vi "data_type_equal.vi"(8 "error in":errorcluster, 10 "Data Cluster":variant, 11 "Stream data cluster":refnum<class "stream_custom_cluster.lvclass">) -> (0 "error out":errorcluster, 2 "dub Data Cluster":variant, 3 "Stream data cluster out":refnum<class "stream_custom_cluster.lvclass">)   [LabVIEW 2020, in "stream_custom_cluster.lvclass"]
uses:
  stream_custom_cluster.lvclass
  stream_custom_cluster.lvclass/stream_custom_cluster.ctl
  <vilib>/Utility/Data Type/NI_Data Type.lvlib
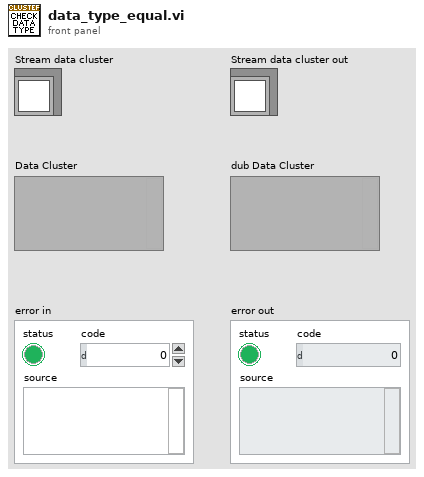
[diagram p1: front panel]
types:
  T1 = typedef "stream_custom_cluster.lvclass/private data.ctl" = cluster{"type":T2[], "channel names":string[], "data":refnum<queue>[], "cluster element types":variant[]}
  T2 = typedef "openg_variant.lvlib/Type Descriptor Enumeration__ogtk.ctl" = enum8{"<Null>", "I8", "I16", "I32", "I64", "U8", "U16", "U32", "U64", "SGL", "DBL", "EXT", "CSG", "CDB", "CXT", "0x0F", "0x10", "0x11", "0x12", "0x13", "0x14", "Enum U8", "Enum U16", "Enum U32", "Enum U64", "SGL PQ", "DBL PQ", "EXT PQ", "CSG PQ", "CDB PQ", "CXT PQ", "0x1F", "0x20", "Boolean", "0x22", "0x23", "0x24", "0x25", "0x26", "0x27", "0x28", "0x29", "0x2A", "0x2B", "0x2C", "0x2D", "0x2E", "0x2F", "String", "0x31", "Path", "Pict", "0x34", "0x35", "0x36", "DAQ", "0x38", "0x39", "0x3A", "0x3B", "0x3C", "0x3D", "0x3E", "0x3F", "Array", "0x41", "0x42", "0x43", "0x44", "0x45", "0x46", "0x47", "0x48", "0x49", "0x4A", "0x4B", "0x4C", "0x4D", "0x4E", "0x4F", "Cluster", "0x51", "0x52", "Variant", "Waveform", "0x55", "0x56", "0x57", "0x58", "0x59", "0x5A", "0x5B", "0x5C", "0x5D", "0x5E", "Fixed Point", "0x60", "0x61", "0x62", "0x63", "0x64", "0x65", "0x66", "0x67", "0x68", "0x69", "0x6A", "0x6B", "0x6C", "0x6D", "0x6E", "0x6F", "Refnum", "0x71", "0x72", "Set Collection", "Map Collection"}
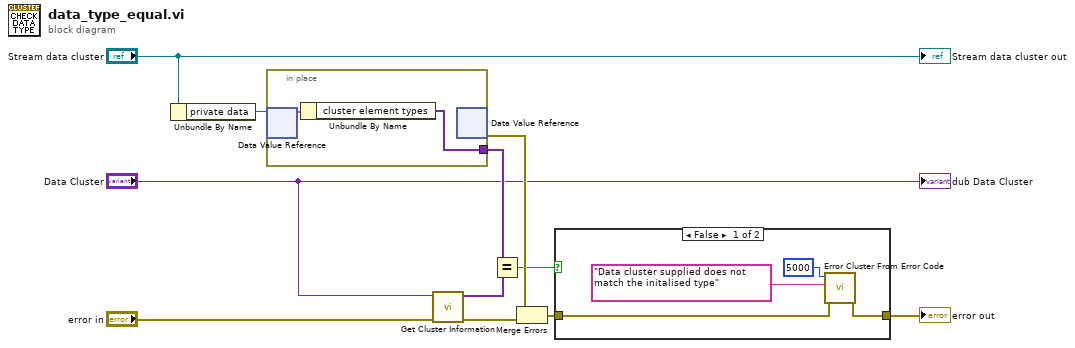
[diagram p0: block diagram]
diagram:
  n1 = Unbundle By Name("Stream data cluster") -> ("private data"=w10:refnum<data-value>)
  n2 = in-place {
    in-place-border: [w12] -> w9
    n3 = in-place-dvr #1(w10) -> (w13:T1)  [unwired: 1 out]
    n4 = Unbundle By Name(w13) -> ("cluster element types"=w12:variant[])
    n5 = in-place-dvr #1() -> (w11:errorcluster)  [unwired: 1 in, 1 out]
  }
  n6 = call <vilib>:"Get Cluster Information.vi"("error in (no error)"="error in", "variant"="Data Cluster") -> ("error out"=w4:errorcluster, "cluster elements"=w8:variant[])  [unwired: 8 in]
  n7 = Equal?(x=w9, y=w8) -> (x = y?=w1:bool)
  n8 = Merge Errors(w11, w4) -> (w3:errorcluster)
  n9 = case shown="False" w1 {
    tunnel: w3 -> [w15 w18]
    tunnel: [w14 w18] -> w2
    frame False {
      n10 = call <vilib>:"Error Cluster From Error Code.vi"("error in (no error)"=w15, "error message (\"\")"="Data cluster supplied does not match the initalised type" ("error message (\"\")"), "error code (0)"=5000) -> ("error out"=w14:errorcluster)  [unwired: 6 in]
    }
    frame True {
    }
  }
  "error out" <- w2
  "dub Data Cluster" <- "Data Cluster"
  "Stream data cluster out" <- "Stream data cluster"
